vi "AdjustXYLegend.vi"(10 "SelectedSigList":refnum<vi>, 11 "XYGraph输入":refnum<vi>) -> ()   [LabVIEW 2015]
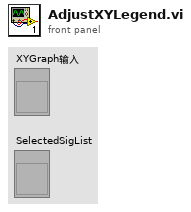
[diagram p1: front panel]
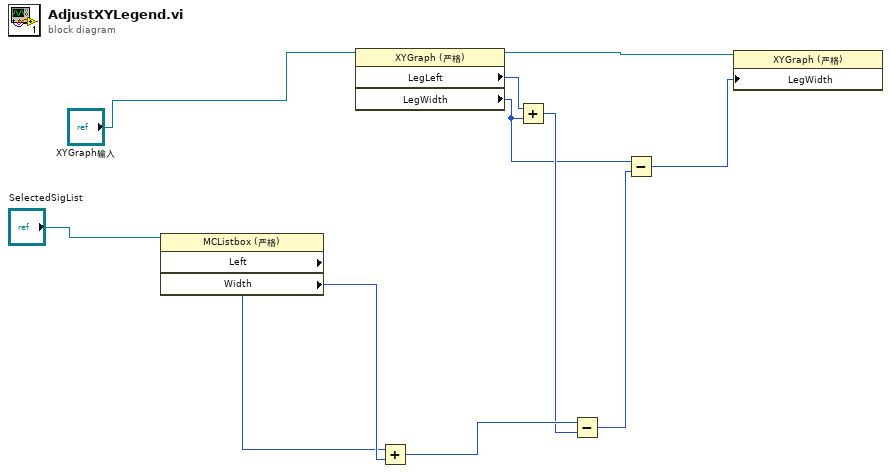
[diagram p0: block diagram]
diagram:
  n1 = property class="MCListbox (严格)"(reference="SelectedSigList") -> ("Left"=w8:i32, "Width"=w9:u32)  [unwired: 1 in, 2 out]
  n2 = property class="XYGraph (严格)"(reference="XYGraph输入") -> (reference out=w11:refnum<vi>, "LegLeft"=w5:i32, "LegWidth"=w3:u32)  [unwired: 1 in, 1 out]
  n3 = Add(x=w8, y=w9) -> (x+y=w6:u32)
  n4 = Add(x=w5, y=w3) -> (x+y=w4:u32)
  n5 = Subtract(x=w6, y=w4) -> (x-y=w2:u32)
  n6 = Subtract(x=w3, y=w2) -> (x-y=w1:u32)
  n7 = property class="XYGraph (严格)"(reference=w11, "LegWidth"=w1) -> ()  [unwired: 1 in, 2 out]
